vi "InitializeOutputs.vi"(8 "error in (no error)":errorcluster, 11 "Highland T564 DDG in":refnum<class "Highland T564 DDG.lvclass">) -> (0 "error out":errorcluster, 3 "Highland T564 DDG out":refnum<class "Highland T564 DDG.lvclass">)   [LabVIEW 2013, in "Highland T564 DDG.lvclass"]
uses:
  Highland T564 DDG.lvclass
  SupportLibraries/DeviceSpecific/HighlandT560Lib/Common/TypeDefs/ChannelName.ctl
  SupportLibraries/DeviceSpecific/HighlandT560Lib/T560OutputClass/T560Output.lvclass
  Highland T564 DDG.lvclass/Highland T564 DDG.ctl
  SupportLibraries/DeviceSpecific/HighlandT560Lib/T560SessionClass/T560Session.lvclass
  SupportLibraries/DeviceSpecific/HighlandT560Lib/T560ChannelClass/T560Channel.lvclass
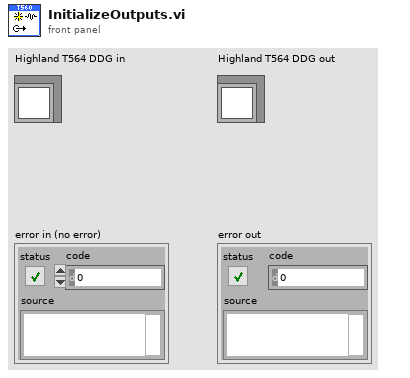
[diagram p1: front panel]
types:
  T1 = typedef "T560Channel.lvclass/ChannelName.ctl" = enum16{"Null", "A", "B", "C", "D", "Trigger"}
  T2 = typedef "Choice83.ctl" = enum16{"Direct", "Inverted"}
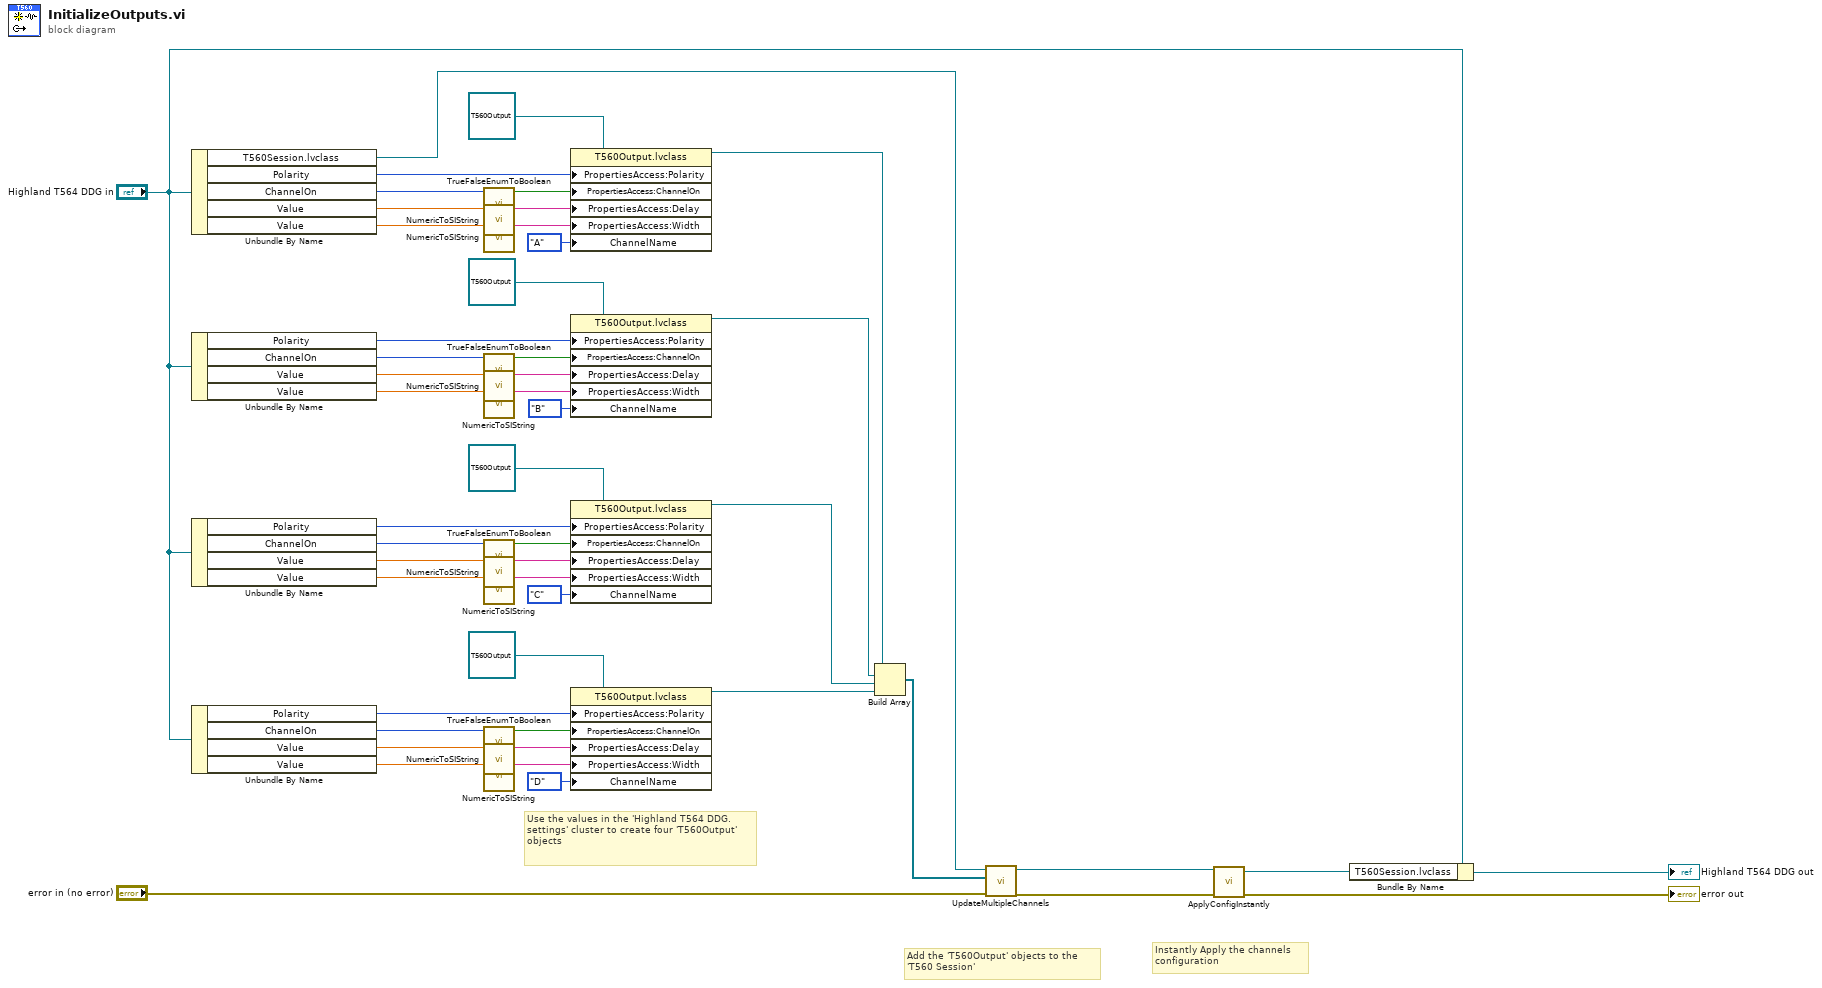
[diagram p0: block diagram]
diagram:
  # "Add the 'T560Output' objects to the \n'T560 Session'"
  # "Use the values in the 'Highland T564 DDG.settings' cluster to create four 'T560Output' objects"
  # "Instantly Apply the channels \nconfiguration"
  n1 = Unbundle By Name("Highland T564 DDG in") -> ("T560Session.lvclass"=w35:refnum<class "T560Session.lvclass">, "Polarity"=w48:T2, "ChannelOn"=w39:enum16{"off", "on"}, "Value"=w47:dbl, "Value"=w46:dbl)
  n2 = Unbundle By Name("Highland T564 DDG in") -> ("Polarity"=w26:T2, "ChannelOn"=w31:enum16{"off", "on"}, "Value"=w27:dbl, "Value"=w28:dbl)
  n3 = Unbundle By Name("Highland T564 DDG in") -> ("Polarity"=w23:T2, "ChannelOn"=w18:enum16{"off", "on"}, "Value"=w22:dbl, "Value"=w21:dbl)
  n4 = Unbundle By Name("Highland T564 DDG in") -> ("Polarity"=w6:T2, "ChannelOn"=w11:enum16{"off", "on"}, "Value"=w7:dbl, "Value"=w8:dbl)
  n5 = call "TrueFalseEnumToBoolean.vi"("ChannelOn"=w39) -> ("selection"=w38:bool)  [unwired: 9 in, 1 out]
  n6 = call "NumericToSIString.vi"("Numeric"=w47) -> ("SI_String"=w37:string)  [unwired: 9 in, 1 out]
  n7 = call "NumericToSIString.vi"("Numeric"=w46) -> ("SI_String"=w36:string)  [unwired: 9 in, 1 out]
  n8 = call "TrueFalseEnumToBoolean.vi"("ChannelOn"=w31) -> ("selection"=w32:bool)  [unwired: 9 in, 1 out]
  n9 = call "NumericToSIString.vi"("Numeric"=w27) -> ("SI_String"=w33:string)  [unwired: 9 in, 1 out]
  n10 = call "NumericToSIString.vi"("Numeric"=w28) -> ("SI_String"=w34:string)  [unwired: 9 in, 1 out]
  n11 = call "TrueFalseEnumToBoolean.vi"("ChannelOn"=w18) -> ("selection"=w17:bool)  [unwired: 9 in, 1 out]
  n12 = call "NumericToSIString.vi"("Numeric"=w22) -> ("SI_String"=w16:string)  [unwired: 9 in, 1 out]
  n13 = call "NumericToSIString.vi"("Numeric"=w21) -> ("SI_String"=w15:string)  [unwired: 9 in, 1 out]
  n14 = call "TrueFalseEnumToBoolean.vi"("ChannelOn"=w11) -> ("selection"=w12:bool)  [unwired: 9 in, 1 out]
  n15 = call "NumericToSIString.vi"("Numeric"=w7) -> ("SI_String"=w13:string)  [unwired: 9 in, 1 out]
  n16 = call "NumericToSIString.vi"("Numeric"=w8) -> ("SI_String"=w14:string)  [unwired: 9 in, 1 out]
  n17 = property class="T560Output.lvclass"(reference=refnum<class "T560Output.lvclass"> refnum ("Highlandt564.lvlib:T560Output.lvclass"), "PropertiesAccess:Polarity"=w48, "PropertiesAccess:ChannelOn"=w38, "PropertiesAccess:Delay"=w37, "PropertiesAccess:Width"=w36, "ChannelName"=ChannelName."A") -> (reference out=w45:refnum<class "T560Output.lvclass">)  [unwired: 1 in, 1 out]
  n18 = property class="T560Output.lvclass"(reference=refnum<class "T560Output.lvclass"> refnum ("Highlandt564.lvlib:T560Output.lvclass"), "PropertiesAccess:Polarity"=w26, "PropertiesAccess:ChannelOn"=w32, "PropertiesAccess:Delay"=w33, "PropertiesAccess:Width"=w34, "ChannelName"=ChannelName."B") -> (reference out=w24:refnum<class "T560Output.lvclass">)  [unwired: 1 in, 1 out]
  n19 = property class="T560Output.lvclass"(reference=refnum<class "T560Output.lvclass"> refnum ("Highlandt564.lvlib:T560Output.lvclass"), "PropertiesAccess:Polarity"=w23, "PropertiesAccess:ChannelOn"=w17, "PropertiesAccess:Delay"=w16, "PropertiesAccess:Width"=w15, "ChannelName"=ChannelName."C") -> (reference out=w4:refnum<class "T560Output.lvclass">)  [unwired: 1 in, 1 out]
  n20 = property class="T560Output.lvclass"(reference=refnum<class "T560Output.lvclass"> refnum ("Highlandt564.lvlib:T560Output.lvclass"), "PropertiesAccess:Polarity"=w6, "PropertiesAccess:ChannelOn"=w12, "PropertiesAccess:Delay"=w13, "PropertiesAccess:Width"=w14, "ChannelName"=ChannelName."D") -> (reference out=w3:refnum<class "T560Output.lvclass">)  [unwired: 1 in, 1 out]
  n21 = Build Array(w45, w24, w4, w3) -> (w25:refnum<class "T560Output.lvclass">[])
  n22 = call-dynamic "UpdateMultipleChannels.vi"("error in (no error)"="error in (no error)", "ChannelsIn"=w25, "T560Session in"=w35) -> ("error out"=w42:errorcluster, "T560Session out"=w44:refnum<class "T560Session.lvclass">)  [unwired: 7 in]
  n23 = call-dynamic "ApplyConfigInstantly.vi"("error in"=w42, "T560Session in"=w44) -> ("error out"=→"error out":errorcluster, "T560Session out"=w43:refnum<class "T560Session.lvclass">)  [unwired: 8 in]
  n24 = Bundle By Name(cluster="Highland T564 DDG in", "T560Session.lvclass"=w43) -> (→"Highland T564 DDG out":refnum<class "Highland T564 DDG.lvclass">)
